vi "Light up fired scintillators.vi"(7 "Hit color":T3, 8 "error in (no error)":errorcluster, 9 "Hits to display":T2, 10 "No hit color":T3, 11 "SceneObject in":refnum<vi>) -> (0 "error out":errorcluster, 3 "SceneObject out":refnum<vi>)   [LabVIEW 2016]
uses:
  <vilib>/Utility/miscctls.llb/LVRGBAColorTypeDef.ctl
  Typedefs/Coincidence.ctl
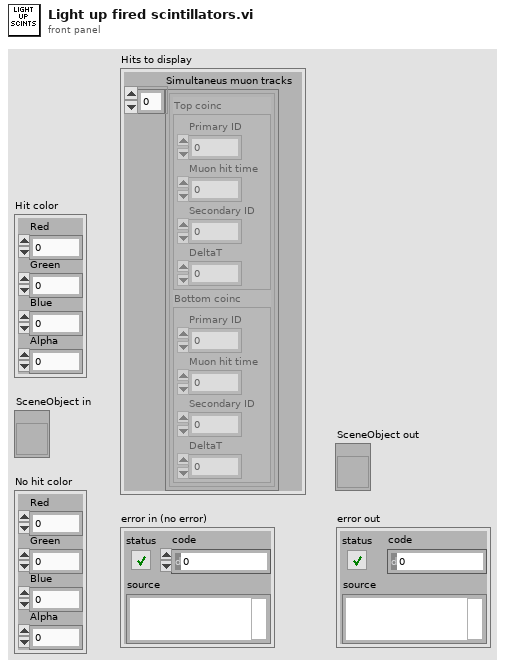
[diagram p1: front panel]
types:
  T1 = typedef "Coincidence.ctl" = cluster{"Primary ID":i8, "Muon hit time":u64, "Secondary ID":i8, "DeltaT":i32}
  T2 = cluster{"Simultaneus muon tracks":cluster{"Top coinc":T1, "Bottom coinc":T1}[]}
  T3 = typedef "LVRGBAColorTypeDef.ctl" = cluster{"Red":sgl, "Green":sgl, "Blue":sgl, "Alpha":sgl}
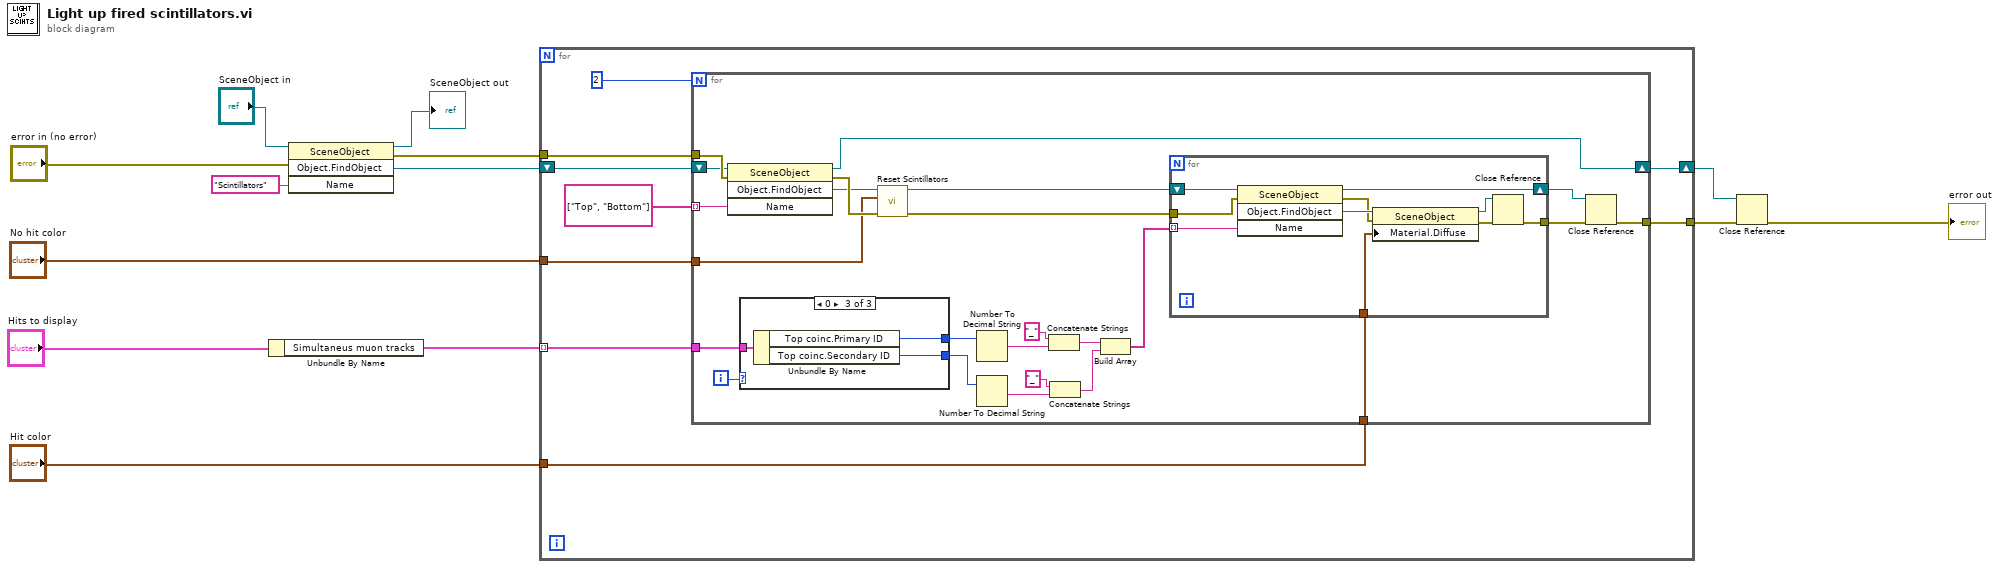
[diagram p0: block diagram]
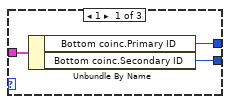
[diagram p2: hidden frame]
diagram:
  n1 = Unbundle By Name("Hits to display") -> ("Simultaneus muon tracks"=w1:cluster{"Top coinc":T1, "Bottom coinc":T1}[])
  n2 = invoke class="SceneObject" method="Object.FindObject"(reference="SceneObject in", error in="error in (no error)", "Name"="Scintillators") -> (reference out=→"SceneObject out":refnum<vi>, error out=w13:errorcluster, "FindObject"=w7:refnum<vi>)  [unwired: 1 in, 1 out]
  n3 = for {
    tunnel: w1 -> [w22] mode=indexing
    tunnel: "Hit color" -> [w21]
    tunnel: "No hit color" -> [w14]
    shift-right: [w18] -> w9
    shift-left: w7 -> [w16]
    tunnel: [w17] -> w8
    tunnel: w13 -> [w15]
    n4 = for {
      N: 2 -> [_]
      tunnel: w22 -> [w46]
      tunnel: w21 -> [w41]
      tunnel: string[] ["Top", "Bottom"] -> [w34] mode=indexing
      shift-right: [w31] -> w18
      shift-left: w16 -> [w28]
      tunnel: [w30] -> w17
      tunnel: w15 -> [w29]
      tunnel: w14 -> [w23]
      i -> [w35]
      n5 = invoke class="SceneObject" method="Object.FindObject"(reference=w28, error in=w29, "Name"=w34) -> (reference out=w31:refnum<vi>, error out=w27:errorcluster, "FindObject"=w26:refnum<vi>)  [unwired: 1 in, 1 out]
      n6 = case shown="0" w35 {
        tunnel: w46 -> [w49 _ w52]
        tunnel: [w48 _ w51] -> w45
        tunnel: [w47 _ w50] -> w44
        frame 1 {
          n7 = Unbundle By Name(w49) -> ("Bottom coinc.Primary ID"=w48:i8, "Bottom coinc.Secondary ID"=w47:i8)
        }
        frame Default {
          # "This case is never entered."
        }
        frame 0 {
          n8 = Unbundle By Name(w52) -> ("Top coinc.Primary ID"=w51:i8, "Top coinc.Secondary ID"=w50:i8)
        }
      }
      n9 = call "Reset Scintillators.vi"("error in (no error)"=w27, "No hit color"=w23, "Scintillator plane in"=w26) -> ("error out"=w24:errorcluster, "Scintillator plane out"=w25:refnum<vi>)  [unwired: 7 in]
      n10 = Number To Decimal String(number=w45) -> (decimal integer string=w42:string)  [unwired: 1 in]
      n11 = Number To Decimal String(number=w44) -> (decimal integer string=w40:string)  [unwired: 1 in]
      n12 = Concatenate Strings("_" ("string"), w42) -> (w38:string)
      n13 = Concatenate Strings("_" ("string"), w40) -> (w37:string)
      n14 = Build Array(w38, w37) -> (w36:string[])
      n15 = for {
        tunnel: w41 -> [w53]
        tunnel: w36 -> [w60] mode=indexing
        shift-right: [w56] -> w32
        shift-left: w25 -> [w62]
        tunnel: [w55] -> w33
        tunnel: w24 -> [w54]
        n16 = invoke class="SceneObject" method="Object.FindObject"(reference=w62, error in=w54, "Name"=w60) -> (reference out=w56:refnum<vi>, error out=w57:errorcluster, "FindObject"=w61:refnum<vi>)  [unwired: 1 in, 1 out]
        n17 = property class="SceneObject"(reference=w61, error in=w57, "Material.Diffuse"=w53) -> (reference out=w58:refnum<vi>, error out=w59:errorcluster)
        n18 = Close Reference(reference=w58, error in (no error)=w59) -> (error out=w55:errorcluster)
      }
      n19 = Close Reference(reference=w32, error in (no error)=w33) -> (error out=w30:errorcluster)
    }
  }
  n20 = Close Reference(reference=w9, error in (no error)=w8) -> (error out=→"error out":errorcluster)
